vi "__PW.vi"(8 "VC(V)":dbl=1.5, 9 "VB(V)":dbl, 10 "VA(V)":dbl=8.0, 11 "GPIB":string="6") -> (0 "ACmoni":dbl, 1 "ABmoni":dbl, 2 "AAmoni":dbl)   [LabVIEW 2017]
panel:
  out "VCmoni":dbl
  in  "AC(A)":dbl=2.5
  out "VBmoni":dbl
  out "VAmoni":dbl
  in  "Wait(ms)":i32
  out "文字列":string="VA1.00,AA2.30,VB0.00,AB0.10"
  in  "AB(A)":dbl=0.1
  in  "AA(A)":dbl=0.9
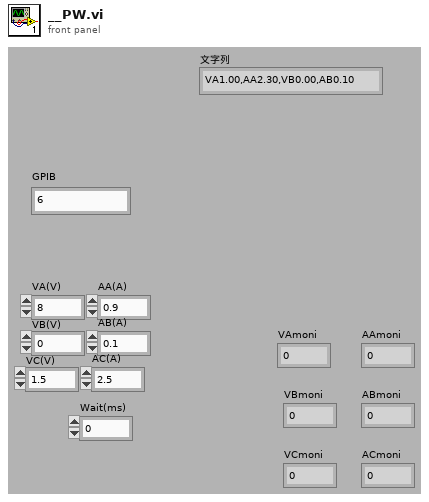
[diagram p1: front panel]
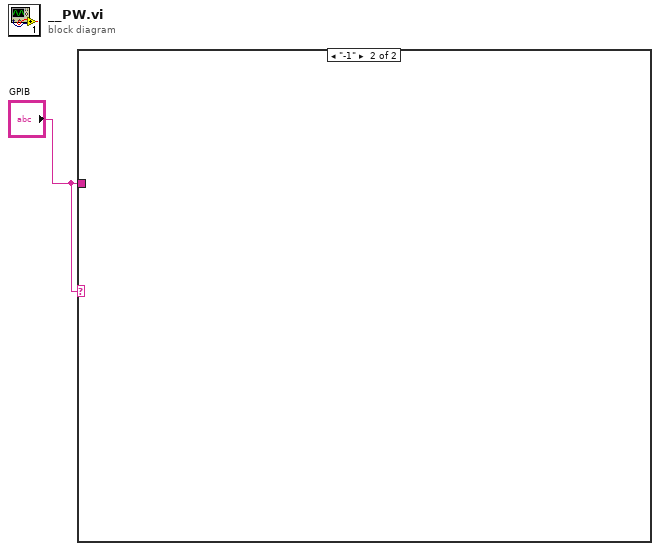
[diagram p0: block diagram]
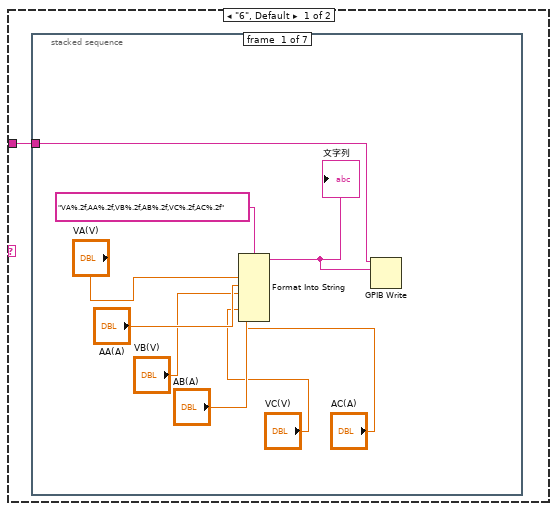
[diagram p2: hidden frame]
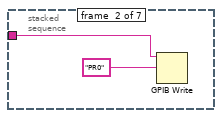
[diagram p3: hidden frame]
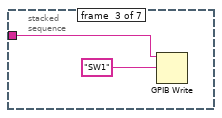
[diagram p4: hidden frame]
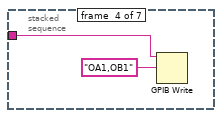
[diagram p5: hidden frame]
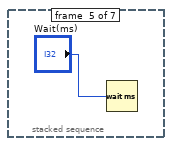
[diagram p6: hidden frame]
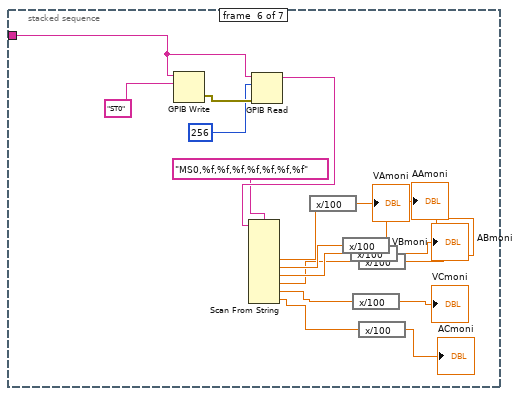
[diagram p7: hidden frame]
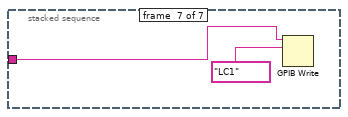
[diagram p8: hidden frame]
diagram:
  n1 = case shown="\"-1\"" "GPIB" {
    tunnel: "GPIB" -> [w2 _]
    frame "6", Default {
      n2 = stacked-sequence {
        tunnel: w2 -> [w6 w13 w15 w17 _ w34 w37]
        frame #0 {
          n3 = Format Into String(format string="VA%.2f,AA%.2f,VB%.2f,AB%.2f,VC%.2f,AC%.2f", "VA(V)", "AA(A)", "VB(V)", "AB(A)", "VC(V)", "AC(A)") -> (resulting string=w5:string)  [unwired: 2 in, 1 out]
          "文字列" <- w5
          n4 = GPIB Write(0:w6, 1:w5) -> ()  [unwired: 3 in, 2 out]
        }
        frame #1 {
          n5 = GPIB Write(0:w13, 1:"PR0") -> ()  [unwired: 3 in, 2 out]
        }
        frame #2 {
          n6 = GPIB Write(0:w15, 1:"SW1") -> ()  [unwired: 3 in, 2 out]
        }
        frame #3 {
          n7 = GPIB Write(0:w17, 1:"OA1,OB1") -> ()  [unwired: 3 in, 2 out]
        }
        frame #4 {
          n8 = Wait (ms)(milliseconds to wait="Wait(ms)") -> ()  [unwired: 1 out]
        }
        frame #5 {
          n9 = GPIB Write(0:w34, 1:"ST0") -> (6:w35:errorcluster)  [unwired: 3 in, 1 out]
          n10 = GPIB Read(0:w34, 1:256, 3:w35) -> (5:w32:string)  [unwired: 2 in, 2 out]
          n11 = Scan From String(format string="MS0,%f,%f,%f,%f,%f,%f,%f", input string=w32) -> (output 2=w29:dbl, output 3=w25:dbl, output 4=w24:dbl, output 5=w23:dbl, output 6=w20:dbl, output 7=w19:dbl)  [unwired: 10 in, 3 out]
          n12 = expression code="x/100"(w29) -> (→"VAmoni":dbl)
          n13 = expression code="x/100"(w25) -> (→"AAmoni":dbl)
          n14 = expression code="x/100"(w24) -> (→"VBmoni":dbl)
          n15 = expression code="x/100"(w20) -> (→"VCmoni":dbl)
          n16 = expression code="x/100"(w23) -> (→"ABmoni":dbl)
          n17 = expression code="x/100"(w19) -> (→"ACmoni":dbl)
        }
        frame #6 {
          n18 = GPIB Write(0:w37, 1:"LC1") -> ()  [unwired: 3 in, 2 out]
        }
      }
    }
    frame "-1" {
    }
  }
